vi "Apply Trim.vi"(8 "Backwards Tuning":T1={"Max Speed"=0.0, "Min Speed"=0.0, "L/R"=FALSE, "Deadzone"=1.0} {"Deadzone" min=0.0 max=1.0; "Min Speed" min=0.0 max=1.0}, 9 "Forward Tuning":T1={"Max Speed"=0.0, "Min Speed"=0.0, "L/R"=FALSE, "Deadzone"=1.0} {"Deadzone" min=0.0 max=1.0; "Min Speed" min=0.0 max=1.0; "Max Speed" min=0.0 max=1.0}, 10 "Speed":dbl, 11 "Turn":dbl) -> (3 "Trimmed Turn":dbl)   [LabVIEW 2016]
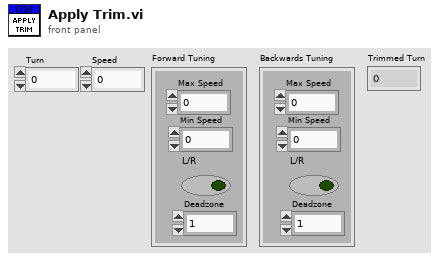
[diagram p1: front panel]
types:
  T1 = cluster{"Max Speed":dbl, "Min Speed":dbl, "L/R":bool, "Deadzone":dbl}
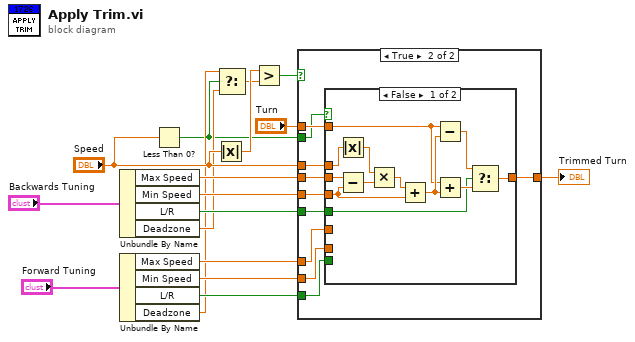
[diagram p0: block diagram]
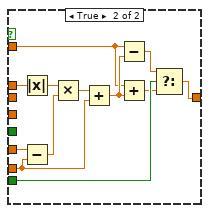
[diagram p3: hidden frame]
diagram:
  n1 = Unbundle By Name("Backwards Tuning") -> ("Max Speed"=w8:dbl, "Min Speed"=w7:dbl, "L/R"=w6:bool, "Deadzone"=w4:dbl)
  n2 = Unbundle By Name("Forward Tuning") -> ("Max Speed"=w16:dbl, "Min Speed"=w15:dbl, "L/R"=w14:bool, "Deadzone"=w3:dbl)
  n3 = Less Than 0?(x="Speed") -> (x < 0?=w1:bool)
  n4 = Absolute Value(x="Speed") -> (abs(x)=w13:dbl)
  n5 = Select(t=w3, s=w1, f=w4) -> (s? t:f=w2:dbl)
  n6 = Greater?(x=w13, y=w2) -> (0:w10:bool)
  n7 = case shown="True" w10 {
    tunnel: w16 -> [_ w28]
    tunnel: w15 -> [_ w23]
    tunnel: w14 -> [_ w27]
    tunnel: "Speed" -> [_ w26]
    tunnel: "Turn" -> [w18 w25]
    tunnel: [w18 w24] -> w11
    tunnel: w8 -> [_ w22]
    tunnel: w7 -> [_ w21]
    tunnel: w6 -> [_ w20]
    tunnel: w1 -> [_ w19]
    frame False {
    }
    frame True {
      n8 = case shown="False" w19 {
        tunnel: w28 -> [_ w52]
        tunnel: w27 -> [_ w50]
        tunnel: w26 -> [w32 w41]
        tunnel: w25 -> [w29 w46]
        tunnel: [w34 w45] -> w24
        tunnel: w23 -> [_ w43]
        tunnel: w22 -> [w31 _]
        tunnel: w21 -> [w30 _]
        tunnel: w20 -> [w33 _]
        frame False {
          n9 = Absolute Value(x=w32) -> (abs(x)=w35:dbl)
          n10 = Subtract(x=w31, y=w30) -> (x-y=w40:dbl)
          n11 = Multiply(x=w35, y=w40) -> (x*y=w36:dbl)
          n12 = Add(x=w36, y=w30) -> (x+y=w38:dbl)
          n13 = Subtract(x=w29, y=w38) -> (x-y=w37:dbl)
          n14 = Add(x=w29, y=w38) -> (x+y=w39:dbl)
          n15 = Select(t=w37, s=w33, f=w39) -> (s? t:f=w34:dbl)
        }
        frame True {
          n16 = Absolute Value(x=w41) -> (abs(x)=w42:dbl)
          n17 = Subtract(x=w52, y=w43) -> (x-y=w51:dbl)
          n18 = Multiply(x=w42, y=w51) -> (x*y=w44:dbl)
          n19 = Add(x=w44, y=w43) -> (x+y=w48:dbl)
          n20 = Subtract(x=w46, y=w48) -> (x-y=w47:dbl)
          n21 = Add(x=w46, y=w48) -> (x+y=w49:dbl)
          n22 = Select(t=w47, s=w50, f=w49) -> (s? t:f=w45:dbl)
        }
      }
    }
  }
  "Trimmed Turn" <- w11
